vi "Load Variable Parameters.vi"(11 "Variant":variant) -> (1 "Node Type":T2, 2 "OPC UA type":T1 items=["Boolean"=1, "SByte"=2, "Byte"=3, "Int16"=4, "UInt16"=5, "Int32"=6, "UInt32"=7, "Int64"=8, "UInt64"=9, "Float"=10, "Double"=11, "String"=12, "DateTime"=13, "ByteString"=15, "Array of Boolean"=101, "Array of SByte"=102, "Array of Byte"=103, "Array of Int16"=104, "Array of UInt16"=105, "Array of Int32"=106, "Array of UInt32"=107, "Array of Int64"=108, "Array of UInt64"=109, "Array of Float"=110, "Array of Double"=111, "Array of String"=112, "Array of DateTime"=113, "Array of ByteString"=115], 3 "SV Data Type":T3, 4 "URL":string)   [LabVIEW 2015]
uses:
  Controls/SV type.ctl
  Controls/Node Type.ctl
  Controls/OPC type.ctl
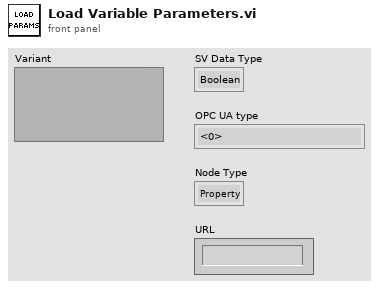
[diagram p1: front panel]
types:
  T1 = typedef "OPC type.ctl" = u16
  T2 = typedef "Node Type.ctl" = enum16{"Property", "Item", "Folder"}
  T3 = typedef "SV type.ctl" = enum16{"Boolean", "SByte", "Byte", "Int16", "UInt16", "Int32", "UInt32", "Int64", "UInt64", "Float", "Double", "String", "DateTime", "ByteString", "Array of Boolean", "Array of SByte", "Array of Byte", "Array of Int16", "Array of UInt16", "Array of Int32", "Array of UInt32", "Array of Int64", "Array of UInt64", "Array of Float", "Array of Double", "Array of String", "Array of DateTime", "Array of ByteString", "Unsupported"}
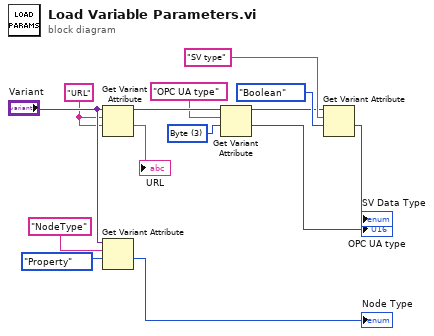
[diagram p0: block diagram]
diagram:
  w4 = T1 3 items=["Boolean"=1, "SByte"=2, "Byte"=3, "Int16"=4, "UInt16"=5, "Int32"=6, "UInt32"=7, "Int64"=8, "UInt64"=9, "Float"=10, "Double"=11, "String"=12, "DateTime"=13, "ByteString"=15, "Array of Boolean"=101, "Array of SByte"=102, "Array of Byte"=103, "Array of Int16"=104, "Array of UInt16"=105, "Array of Int32"=106, "Array of UInt32"=107, "Array of Int64"=108, "Array of UInt64"=109, "Array of Float"=110, "Array of Double"=111, "Array of String"=112, "Array of DateTime"=113, "Array of ByteString"=115] ("OPC type")
  w3 = "URL" ("name")
  n1 = Get Variant Attribute(Variant="Variant", name=w3, default value (empty Variant)=w3) -> (duplicate Variant=w2:variant, value=→"URL":string)  [unwired: 1 in, 2 out]
  n2 = Get Variant Attribute(Variant="Variant", name="NodeType", default value (empty Variant)=Node_Type."Property" ("Node Type")) -> (value=→"Node Type":T2)  [unwired: 1 in, 3 out]
  n3 = Get Variant Attribute(Variant=w2, name="OPC UA type", default value (empty Variant)=w4) -> (duplicate Variant=w11:variant, value=→"OPC UA type":T1)  [unwired: 1 in, 2 out]
  n4 = Get Variant Attribute(Variant=w11, name="SV type", default value (empty Variant)=SV_type."Boolean" ("data type out")) -> (value=→"SV Data Type":T3)  [unwired: 1 in, 3 out]
